vi "_Log Events.vi"(4 "File Name":string, 5 "Log Path":path, 6 "error in (no error)":errorcluster, 7 "Event":string, 8 "time format string (%c)":string="%y/%m/%d; %H:%M:%S%3u", 9 "Log Command":T1) -> (0 "error out":errorcluster, 3 ">10MB":bool)   [LabVIEW 2015]
doc: "This vi maintains a datalog file for plate positions in motor steps.\nEach datalog record consists of the following data members:\nData/time in secs from 12am 1/1/1904.\nHorizontal motor steps\nVertical motor steps\nAll numbers are stored as 8-byte doubles."
uses:
  Type/_Log Command.ctl
  <userlib>/_OpenG.lib/file/file.llb/Strip Path Extension - String__ogtk.vi
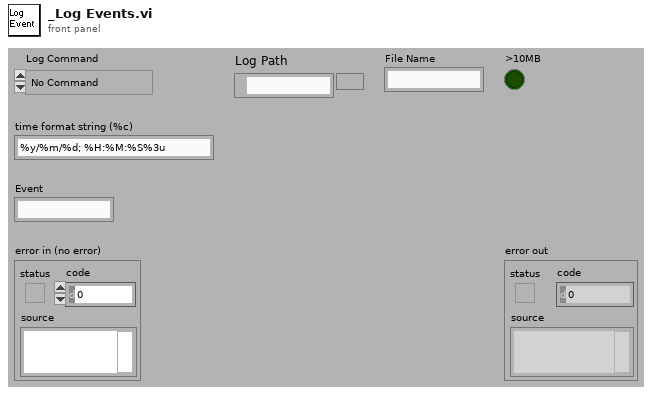
[diagram p1: front panel]
types:
  T1 = typedef "_Log Command.ctl" = enum16{"No Command", "Open", "Read", "Write", "Close", "Check Size"}
  T2 = enum16{"open", "replace", "create", "open or create", "replace or create", "replace or create with confirmation"}
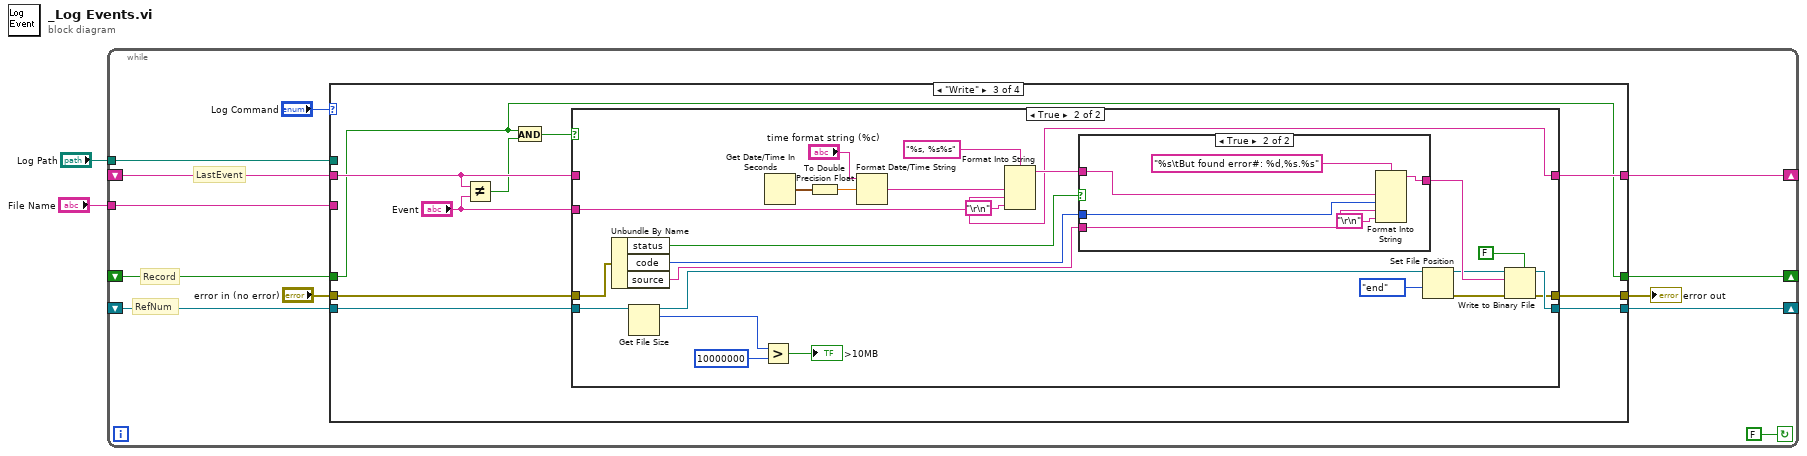
[diagram p0: block diagram]
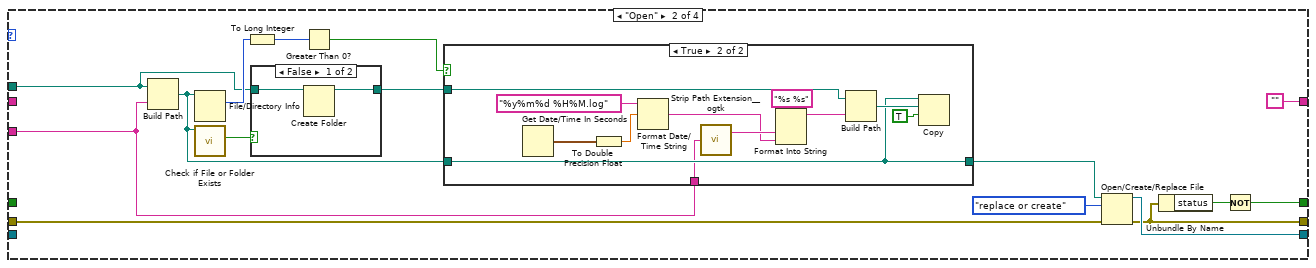
[diagram p3: hidden frame]
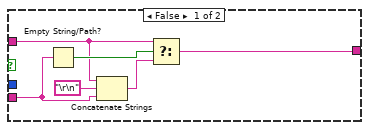
[diagram p7: hidden frame]
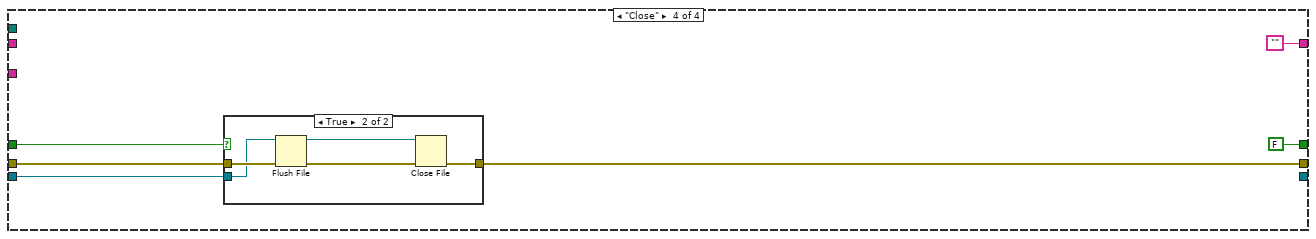
[diagram p8: hidden frame]
diagram:
  n1 = while {
    shift-left: _ -> [w9]
    shift-right: [w10] -> _
    shift-left: _ -> [w11]
    shift-right: [w12] -> _
    shift-right: [w6] -> _
    shift-left: _ -> [w5]
    tunnel: "Log Path" -> [w4]
    tunnel: "File Name" -> [w3]
    stop <- FALSE continue-if-true
    # "Record"
    # "LastEvent"
    # "RefNum"
    n2 = case shown="\"Write\"" "Log Command" {
      tunnel: [w18 w28 w59 _] -> w12
      tunnel: w11 -> [w18 _ w60 w103]
      tunnel: [w17 w33 w52 FALSE ("Record")] -> w10
      tunnel: w9 -> [w17 _ w52 w104]
      tunnel: "error in (no error)" -> [w16 w25 w58 w102]
      tunnel: [w16 w26 w57 w101] -> w7
      tunnel: [w15 "" w56 ""] -> w6
      tunnel: w5 -> [w15 _ w54 _]
      tunnel: w4 -> [_ w23 _ _]
      tunnel: w3 -> [_ w19 _ _]
      frame "No Command", Default {
      }
      frame "Open" {
        n3 = Build Path(base path=w23, name or relative path=w19) -> (appended path=w20:path)
        n4 = File/Directory Info(path=w20) -> (size=w31:i64)  [unwired: 1 in, 6 out]
        n5 = call <vilib>:"Check if File or Folder Exists.vi"("path"=w20) -> ("file or folder exists?"=w21:bool)  [unwired: 8 in, 2 out]
        n6 = To Long Integer(number=w31) -> (32bit integer=w32:i32)
        n7 = case shown="False" w21 {
          tunnel: w23 -> [w36 w37]
          tunnel: [w35 w37] -> w22
          frame False {
            n8 = Create Folder(path (use dialog)=w36) -> (created path=w35:path)  [unwired: 2 in, 2 out]
          }
          frame True {
          }
        }
        n9 = Greater Than 0?(x=w32) -> (x > 0?=w30:bool)
        n10 = case shown="True" w30 {
          tunnel: w20 -> [w38 w44]
          tunnel: w22 -> [_ w50]
          tunnel: [w38 w44] -> w29
          tunnel: w19 -> [_ w42]
          frame False {
          }
          frame True {
            n11 = Get Date/Time In Seconds() -> (seconds since 1Jan1904=w48:timestamp)
            n12 = To Double Precision Float(number=w48) -> (double precision float=w49:dbl)
            n13 = Format Date/Time String(time format string (%c)="%y%m%d %H%M.log", seconds (now)=w49) -> (date/time string=w39:string)  [unwired: 1 out]
            n14 = call-poly <userlib>:"Strip Path Extension__ogtk.vi"("path"=w42) -> ("root"=w41:string)  [unwired: 1 out]
            n15 = Format Into String(format string="%s %s", w41, w39) -> (resulting string=w40:string)  [unwired: 2 in, 1 out]
            n16 = Build Path(base path=w50, name or relative path=w40) -> (appended path=w46:path)
            n17 = Copy(9:TRUE ("overwrite (F)"), 10:w46, 11:w44) -> ()  [unwired: 1 in, 4 out]
          }
        }
        n18 = Open/Create/Replace File(file path (use dialog)=w29, error in=w25, operation (0:open)=T2."replace or create") -> (refnum out=w28:refnum<file>, error out=w26:errorcluster)  [unwired: 3 in, 1 out]
        n19 = Unbundle By Name(w26) -> ("status"=w34:bool)
        n20 = Not(x=w34) -> (.not. x?=w33:bool)
      }
      frame "Write" {
        n21 = Not Equal?(x=w54, y="Event") -> (x != y?=w51:bool)
        n22 = And(x=w52, y=w51) -> (x .and. y?=w53:bool)
        n23 = case shown="True" w53 {
          tunnel: w60 -> [w63 w68]
          tunnel: [w63 w87] -> w59
          tunnel: w58 -> [w62 w75]
          tunnel: [w62 w74] -> w57
          tunnel: [w61 w69] -> w56
          tunnel: w54 -> [w61 _]
          tunnel: "Event" -> [_ w69]
          frame False {
          }
          frame True {
            n24 = Unbundle By Name(w75) -> ("status"=w81:bool, "code"=w80:i32, "source"=w70:string)
            n25 = Get File Size(file=w68) -> (refnum out=w67:refnum<file>, size (in bytes)=w66:i64)  [unwired: 1 in, 1 out]
            n26 = Greater?(x=w66, y=i64 10000000) -> (0:→">10MB":bool)
            n27 = Get Date/Time In Seconds() -> (seconds since 1Jan1904=w77:timestamp)
            n28 = To Double Precision Float(number=w77) -> (double precision float=w86:dbl)
            n29 = Format Date/Time String(time format string (%c)="time format string (%c)", seconds (now)=w86) -> (date/time string=w84:string)  [unwired: 1 out]
            n30 = Format Into String(format string="%s, %s%s" ("Format String"), w84, w69, "\r\n") -> (resulting string=w79:string)  [unwired: 2 in, 1 out]
            n31 = case shown="True" w81 {
              tunnel: w80 -> [_ w99]
              tunnel: w79 -> [w91 w98]
              tunnel: [w88 w96] -> w78
              tunnel: w70 -> [w89 w95]
              frame False {
                n32 = Empty String/Path?(string/path=w89) -> (empty?=w93:bool)
                n33 = Concatenate Strings(w91, "\r\n", w89) -> (w92:string)
                n34 = Select(t=w91, s=w93, f=w92) -> (s? t:f=w88:string)
              }
              frame True {
                n35 = Format Into String(format string="%s\tBut found error#: %d,%s.%s" ("Format String"), w98, w99, w95, "\r\n") -> (resulting string=w96:string)  [unwired: 2 in, 1 out]
              }
            }
            n36 = Set File Position(refnum=w67, from (0:start)=enum16{"start", "end", "current"}."end" ("pos mode (0:2)")) -> (refnum out=w73:refnum<file>, error out=w72:errorcluster)  [unwired: 1 in, 1 out]
            n37 = Write to Binary File(file (use dialog)=w73, data=w78, error in=w72, 5:FALSE ("prepend array or string size? (T)")) -> (refnum out=w87:refnum<file>, error out=w74:errorcluster)  [unwired: 3 out]
          }
        }
      }
      frame "Close" {
        n38 = case shown="True" w104 {
          tunnel: w103 -> [_ w108]
          tunnel: w102 -> [w106 w110]
          tunnel: [w106 w111] -> w101
          frame False {
          }
          frame True {
            n39 = Flush File(refnum=w108, error in=w110) -> (refnum out=w107:refnum<file>, error out=w109:errorcluster)
            n40 = Close File(refnum=w107, error in=w109) -> (error out=w111:errorcluster)  [unwired: 1 out]
          }
        }
      }
    }
    "error out" <- w7
  }
